vi "Validate_EXE_Uninstall.vi"(8 "error in (no error)":errorcluster, 11 "Installer in":refnum<class "Installer.lvclass">) -> (0 "error out":errorcluster, 3 "Installer out":refnum<class "Installer.lvclass">)   [LabVIEW 2020, in "Installer.lvclass"]
uses:
  <vilib>/AppBuilder/IB_Classes/Installer/Installer.lvclass
  <vilib>/AppBuilder/IB_Classes/Installer/Installer.lvclass/Installer.ctl
  <vilib>/AppBuilder/IB_Classes/Source/File/IB_Source_File.lvclass
  <vilib>/AppBuilder/IB_Classes/Source/IB_Source.lvclass
  e:/builds/penguin/labview/branches/2020/dev/dist/vi.lib/AppBuilder/IB_Classes/Source/IB_Source.lvclass
  e:/builds/penguin/labview/branches/2020/dev/dist/vi.lib/AppBuilder/IB_Classes/Source/File/IB_Source_File.lvclass
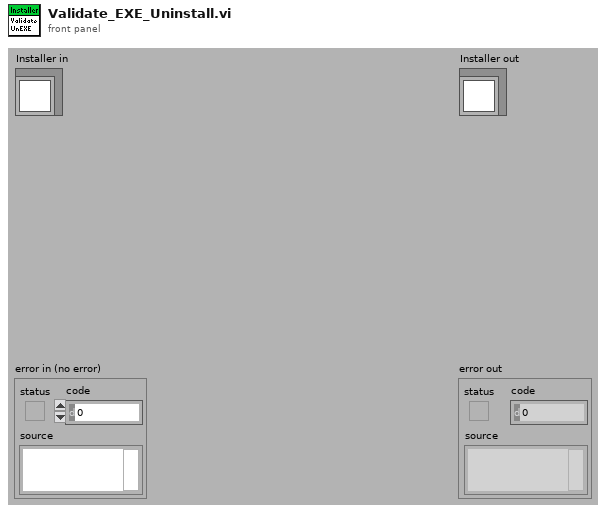
[diagram p1: front panel]
types:
  T1 = typedef "CDK_sTypeDef_FileList.ctl" = cluster{"FileInventory":refnum<class "IB_Source_File.lvclass">, "containerID":string}
  T2 = typedef "IB_Source_File.ctl" = cluster{"Attributes":i16, "RegCOM":bool, "unlock":bool, "shortcuts":refnum<class "IB_Shortcut.lvclass">[], "EXE_install":bool, "CmdArg_install":string, "EXE_uninstall":bool, "CmdArg_uninstall":string}
  T3 = typedef "IB_Source.ctl" = cluster{"name":string, "sourceTag":string, "destTag":string, "path":path, "eng_installPath":string, "UI_inBuild?":bool, "str ref?":bool}
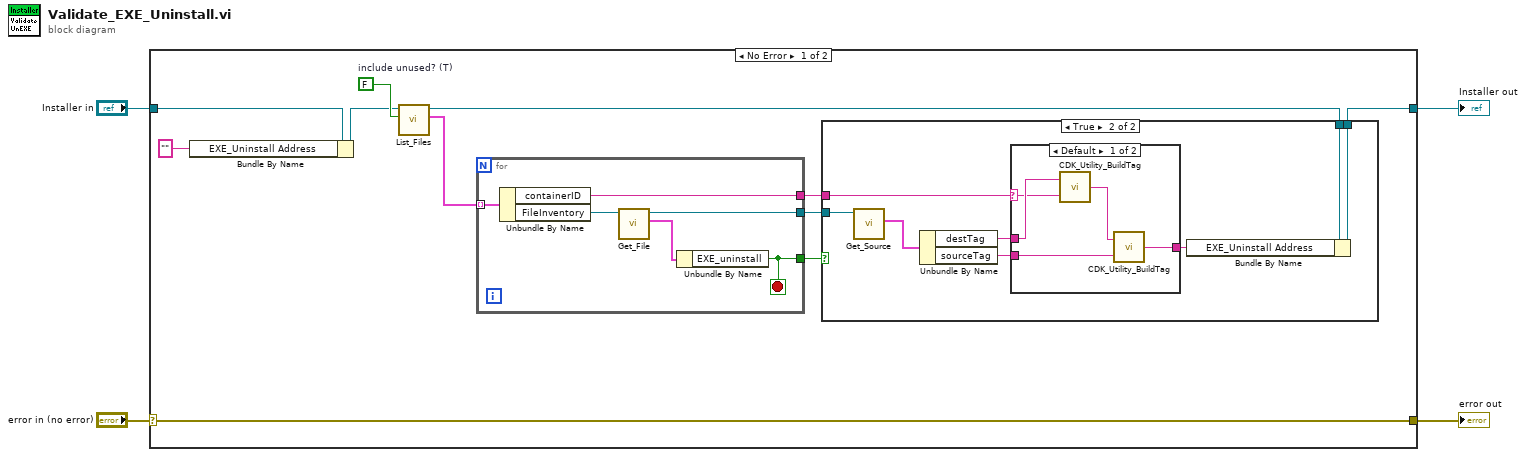
[diagram p0: block diagram]
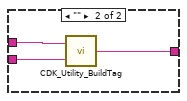
[diagram p3: hidden frame]
diagram:
  n1 = case shown="No Error" "error in (no error)" {
    selector: "error in (no error)" -> [w15 w40]
    tunnel: [w15 w40] -> w3
    tunnel: [w12 w39] -> w1
    tunnel: "Installer in" -> [w6 w39]
    frame No Error {
      w8 = FALSE  # include unused? (T)
      n2 = Bundle By Name(cluster=w6, "EXE_Uninstall Address"="" ("data.exeAddress")) -> (w5:refnum<class "Installer.lvclass">)
      n3 = call <vilib>:"List_Files.vi"("include unused? (T)"=w8, "Installer in"=w5) -> ("files"=w14:T1[], "Installer out"=w13:refnum<class "Installer.lvclass">)  [unwired: 1 in, 7 out]
      n4 = for {
        tunnel: w14 -> [w35] mode=indexing
        tunnel: [w37] -> w10
        tunnel: [w36] -> w11
        tunnel: [w33] -> w9
        stop <- w36 stop-if-true
        n5 = Unbundle By Name(w35) -> ("containerID"=w33:string, "FileInventory"=w34:refnum<class "IB_Source_File.lvclass">)
        n6 = call <vilib>:"Get_File.vi"("IB_Source_File in"=w34) -> ("data"=w38:T2, "IB_Source_File out"=w37:refnum<class "IB_Source_File.lvclass">)  [unwired: 1 in, 8 out]
        n7 = Unbundle By Name(w38) -> ("EXE_uninstall"=w36:bool)
      }
      n8 = case shown="True" w11 {
        tunnel: w13 -> [w16 w24]
        tunnel: [w16 w23] -> w12
        tunnel: w10 -> [_ w21]
        tunnel: w9 -> [_ w18]
        frame False {
        }
        frame True {
          n9 = call <vilib>:"Get_Source.vi"("IB_Source in"=w21) -> ("data"=w22:T3)  [unwired: 1 in, 9 out]
          n10 = Unbundle By Name(w22) -> ("destTag"=w20:string, "sourceTag"=w19:string)
          n11 = case shown="Default" w18 {
            selector: w18 -> [w28 _]
            tunnel: w20 -> [w29 w32]
            tunnel: w19 -> [w26 w31]
            tunnel: [w25 w30] -> w17
            frame Default {
              n12 = call <resource>:"CDK_Utility_BuildTag.vi"("name or relative path"=w28, "BasePath"=w29) -> ("appended path"=w27:string)
              n13 = call <resource>:"CDK_Utility_BuildTag.vi"("name or relative path"=w26, "BasePath"=w27) -> ("appended path"=w25:string)
            }
            frame "" {
              n14 = call <resource>:"CDK_Utility_BuildTag.vi"("name or relative path"=w31, "BasePath"=w32) -> ("appended path"=w30:string)
            }
          }
          n15 = Bundle By Name(cluster=w24, "EXE_Uninstall Address"=w17) -> (w23:refnum<class "Installer.lvclass">)
        }
      }
    }
    frame Error {
    }
  }
  "error out" <- w3
  "Installer out" <- w1
